vi "Parse CfgTable.vi"(7 "Cluster Configuration Typedef":variant, 8 "error in (no error)":errorcluster, 11 "CfgTable Row":string[](array[string])) -> (0 "error out":errorcluster, 1 "Elements":i32, 3 "Cluster Configuration Out":variant)   [LabVIEW 2017, in "ClusterCfgTable.lvlib"]
doc: "Parses a configuration table back into the cluster described by Cluster Configuration Typedef. It is the simple entry point to Parse CfgTable(with DataName).vi."
uses:
  ClusterCfgTable.lvlib
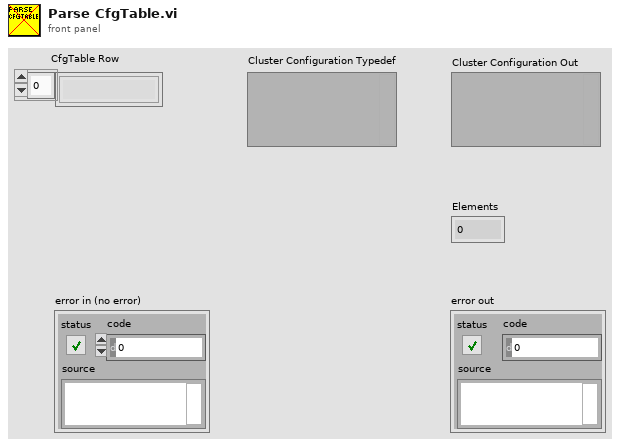
[diagram p1: front panel]
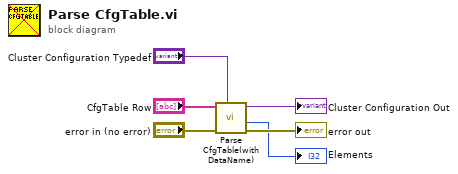
[diagram p0: block diagram]
diagram:
  n1 = call "Parse CfgTable(with DataName).vi"("Cluster Configuration Typedef"="Cluster Configuration Typedef", "error in (no error)"="error in (no error)", "CfgTable Row"="CfgTable Row") -> ("error out"=→"error out":errorcluster, "Elements"=→"Elements":i32, "Cluster Configuration Out"=→"Cluster Configuration Out":variant)  [unwired: 6 in]
